vi "RichToFlatgoogle_protobuf_Type.vi"(5 "OutputClusterType":T1, 11 "InputCluster":T9) -> (3 "OutputCluster":T1)   [LabVIEW 2021, in "NI Measurement V2 Client.lvlib"]
uses:
  NI Measurement V2 Client.lvlib
  google_protobuf_Type.ctl
  google_protobuf_Field.ctl
  google_protobuf_Field_Kind.ctl
  google_protobuf_Field_Cardinality.ctl
  google_protobuf_Option.ctl
  google_protobuf_Any.ctl
  google_protobuf_SourceContext.ctl
  google_protobuf_Syntax.ctl
  google_protobuf_Type_Flat.ctl
  google_protobuf_Field_Flat.ctl
  google_protobuf_Option_Flat.ctl
  google_protobuf_Any_Flat.ctl
  google_protobuf_SourceContext_Flat.ctl
  RichToFlatgoogle_protobuf_Any.vi
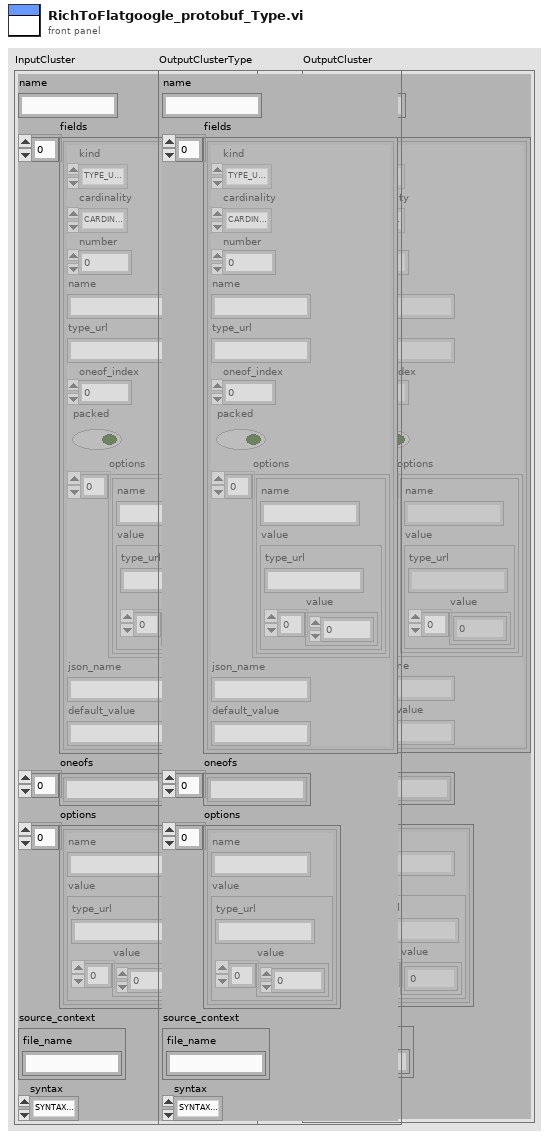
[diagram p1: front panel]
types:
  T1 = typedef "NI Measurement V2 Client.lvlib/google_protobuf_Type_Flat.ctl" = cluster{"name":string, "fields":T2[], "oneofs":string[], "options":T5[], "source_context":T7, "syntax":T8}
  T2 = typedef "NI Measurement V2 Client.lvlib/google_protobuf_Field_Flat.ctl" = cluster{"kind":T3, "cardinality":T4, "number":i32, "name":string, "type_url":string, "oneof_index":i32, "packed":bool, "options":T5[], "json_name":string, "default_value":string}
  T3 = typedef "NI Measurement V2 Client.lvlib/google_protobuf_Field_Kind.ctl" = enum32{"TYPE_UNKNOWN", "TYPE_DOUBLE", "TYPE_FLOAT", "TYPE_INT64", "TYPE_UINT64", "TYPE_INT32", "TYPE_FIXED64", "TYPE_FIXED32", "TYPE_BOOL", "TYPE_STRING", "TYPE_GROUP", "TYPE_MESSAGE", "TYPE_BYTES", "TYPE_UINT32", "TYPE_ENUM", "TYPE_SFIXED32", "TYPE_SFIXED64", "TYPE_SINT32", "TYPE_SINT64"}
  T4 = typedef "NI Measurement V2 Client.lvlib/google_protobuf_Field_Cardinality.ctl" = enum32{"CARDINALITY_UNKNOWN", "CARDINALITY_OPTIONAL", "CARDINALITY_REQUIRED", "CARDINALITY_REPEATED"}
  T5 = typedef "NI Measurement V2 Client.lvlib/google_protobuf_Option_Flat.ctl" = cluster{"name":string, "value":T6}
  T6 = typedef "NI Measurement V2 Client.lvlib/google_protobuf_Any_Flat.ctl" = cluster{"type_url":string, "value":u8[]}
  T7 = typedef "NI Measurement V2 Client.lvlib/google_protobuf_SourceContext_Flat.ctl" = cluster{"file_name":string}
  T8 = typedef "NI Measurement V2 Client.lvlib/google_protobuf_Syntax.ctl" = enum32{"SYNTAX_PROTO2", "SYNTAX_PROTO3"}
  T9 = typedef "NI Measurement V2 Client.lvlib/google_protobuf_Type.ctl" = cluster{"name":string, "fields":T10[], "oneofs":string[], "options":T11[], "source_context":T13, "syntax":T8}
  T10 = typedef "NI Measurement V2 Client.lvlib/google_protobuf_Field.ctl" = cluster{"kind":T3, "cardinality":T4, "number":i32, "name":string, "type_url":string, "oneof_index":i32, "packed":bool, "options":T11[], "json_name":string, "default_value":string}
  T11 = typedef "NI Measurement V2 Client.lvlib/google_protobuf_Option.ctl" = cluster{"name":string, "value":T12}
  T12 = typedef "NI Measurement V2 Client.lvlib/google_protobuf_Any.ctl" = cluster{"type_url":string, "value":u8[]}
  T13 = typedef "NI Measurement V2 Client.lvlib/google_protobuf_SourceContext.ctl" = cluster{"file_name":string}
  T14 = typedef "Measurement Service Client V2.lvlib/google_protobuf_Option_Flat.ctl" = cluster{"name":string, "value":T15}
  T15 = typedef "Measurement Service Client V2.lvlib/google_protobuf_Any_Flat.ctl" = cluster{"type_url":string, "value":u8[]}
  T16 = typedef "Measurement Service Client V2.lvlib/google_protobuf_Field_Flat.ctl" = cluster{"kind":T17, "cardinality":T18, "number":i32, "name":string, "type_url":string, "oneof_index":i32, "packed":bool, "options":T14[], "json_name":string, "default_value":string}
  T17 = typedef "Measurement Service Client V2.lvlib/google_protobuf_Field_Kind.ctl" = enum32{"TYPE_UNKNOWN", "TYPE_DOUBLE", "TYPE_FLOAT", "TYPE_INT64", "TYPE_UINT64", "TYPE_INT32", "TYPE_FIXED64", "TYPE_FIXED32", "TYPE_BOOL", "TYPE_STRING", "TYPE_GROUP", "TYPE_MESSAGE", "TYPE_BYTES", "TYPE_UINT32", "TYPE_ENUM", "TYPE_SFIXED32", "TYPE_SFIXED64", "TYPE_SINT32", "TYPE_SINT64"}
  T18 = typedef "Measurement Service Client V2.lvlib/google_protobuf_Field_Cardinality.ctl" = enum32{"CARDINALITY_UNKNOWN", "CARDINALITY_OPTIONAL", "CARDINALITY_REQUIRED", "CARDINALITY_REPEATED"}
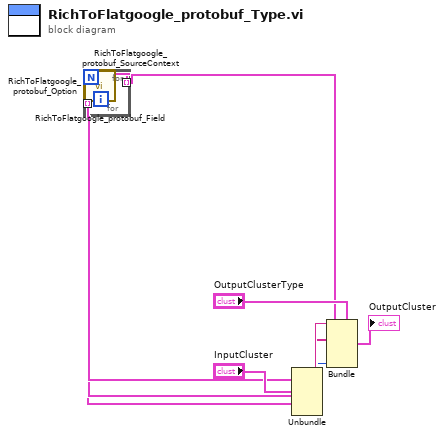
[diagram p0: block diagram]
diagram:
  n1 = Unbundle "Unbundle"("InputCluster") -> ("name"=w9:string, "fields"=w8:T10[], "oneofs"=w6:string[], "options"=w5:T11[], "source_context"=w3:T13, "syntax"=w1:T8)
  n2 = call "RichToFlatgoogle_protobuf_SourceContext.vi"("InputCluster"=w3) -> ("OutputCluster"=w2:T7)  [unwired: 10 in]
  n3 = for {
    tunnel: w5 -> [w14] mode=indexing
    tunnel: [w13] -> w4 mode=indexing
    n4 = call "RichToFlatgoogle_protobuf_Option.vi"("InputCluster"=w14) -> ("OutputCluster"=w13:T14)  [unwired: 10 in]
  }
  n5 = for {
    tunnel: w8 -> [w16] mode=indexing
    tunnel: [w15] -> w7 mode=indexing
    n6 = call "RichToFlatgoogle_protobuf_Field.vi"("InputCluster"=w16) -> ("OutputCluster"=w15:T16)  [unwired: 10 in]
  }
  n7 = Bundle "Bundle"(cluster="OutputClusterType", "name"=w9, "fields"=w7, "oneofs"=w6, "options"=w4, "source_context"=w2, "syntax"=w1) -> (→"OutputCluster":T1)
